vi "FormConfGeral.vi"() -> ()   [LabVIEW 2014]
panel:
  in  "nCycleEdit 6":fxp<+,8,10> caption="Limite inferior (km/h)" format="%#_1f"
  in  "nCycleEdit 5":fxp<+,8,10> caption="Limite superior (km/h)" format="%#_1f"
  in  "nCycleEdit 4":fxp<+,8,10> caption="Tempo entre ciclos (s)" format="%#.0f"
  in  "saveButton":bool
  in  "loadButton":bool
  in  "gainTermoAEdit  18":fxp<+,10,10> caption="Constante (K)"
  in  "gainTermoAEdit  17":fxp<+,10,10> caption="Fator (K)"
  in  "gainTermoAEdit  16":fxp<+,10,10> caption="Fator (K)"
  in  "gainTermoAEdit  15":fxp<+,10,10> caption="Fator (K)"
  in  "gainTermoAEdit  14":fxp<+,10,10> caption="Fator (K)"
  in  "gainTermoAEdit  13":i32 caption="Fator (K)"
  in  "gainTermoAEdit  12":fxp<+,10,10> caption="Limiar"
  in  "gainTermoAEdit  11":fxp<+,10,10> caption="Limiar"
  in  "gainTermoAEdit  10":fxp<+,10,10> caption="Limiar"
  in  "gainTermoAEdit  9":fxp<+,10,10> caption="Limiar"
  in  "gainTermoAEdit  8":fxp<+,10,10> caption="Limiar"
  in  "gainTermoAEdit  7":fxp<+,1,1> caption="Limiar" format="%b"
  in  "Path":path caption="Arquivo de Log"
  in  "nCycleEdit":fxp<+,10,10>=1.0 caption="Número de Ciclos" format="%#_1f"
  # "Configurações Gerais"
  # "Configurações do Ensaio"
  # "Termopar 1"
  # "Termopar 2"
  # "Termopar Ref"
  # "Célula"
  # "Rotação"
  # "Vibração"
  # "Configurações Gerais"
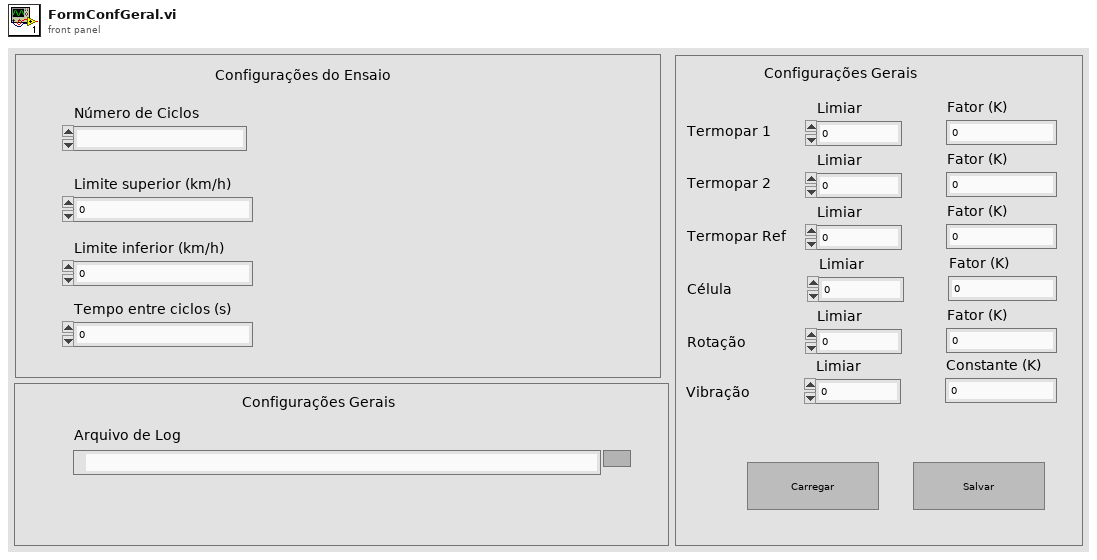
[diagram p1: front panel]
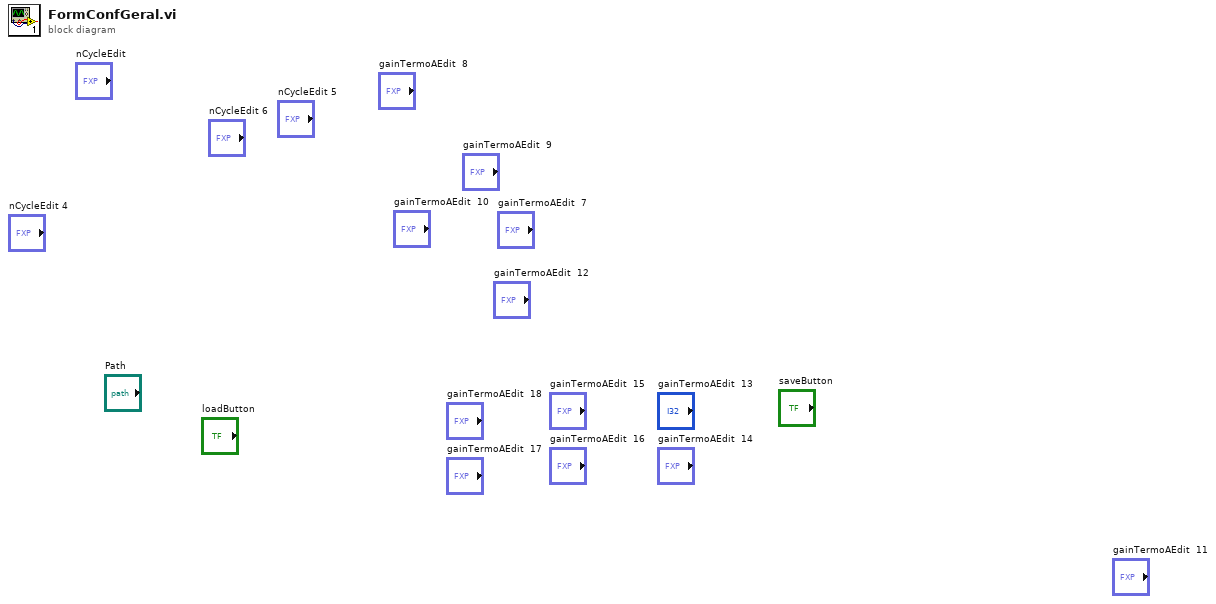
[diagram p0: block diagram]
diagram:
